vi "Access Any.vi"(8 "error in (no error)":errorcluster, 10 "Key":string, 11 "FlexWorktable in":refnum<class "FlexWorktable.lvclass">) -> (0 "error out":errorcluster, 1 "Type":string, 2 "Items out":T1, 3 "FlexWorktable out":refnum<class "FlexWorktable.lvclass">)   [LabVIEW 2022 SP3, in "FlexWorktable.lvclass"]
uses:
  FlexWorktable.lvclass
  Orient3d Class/Orient3d.lvclass
  Vec3d Class/Vec3d.lvclass
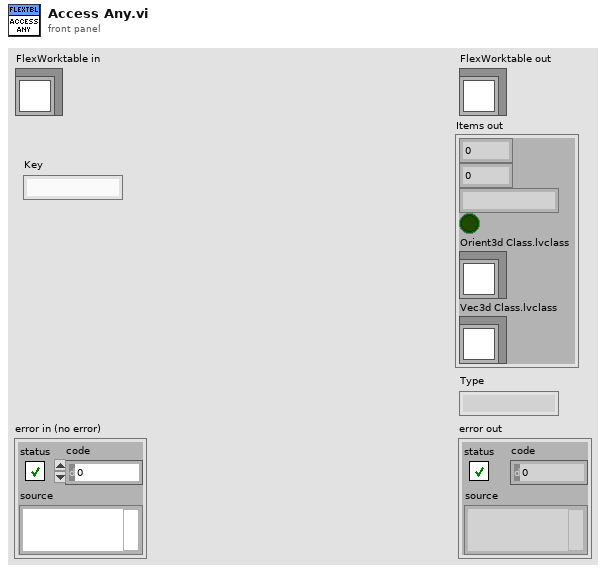
[diagram p1: front panel]
types:
  T1 = cluster{i32, dbl, string, bool, "Orient3d Class.lvclass":refnum<class "Orient3d.lvclass">, "Vec3d Class.lvclass":refnum<class "Vec3d.lvclass">}
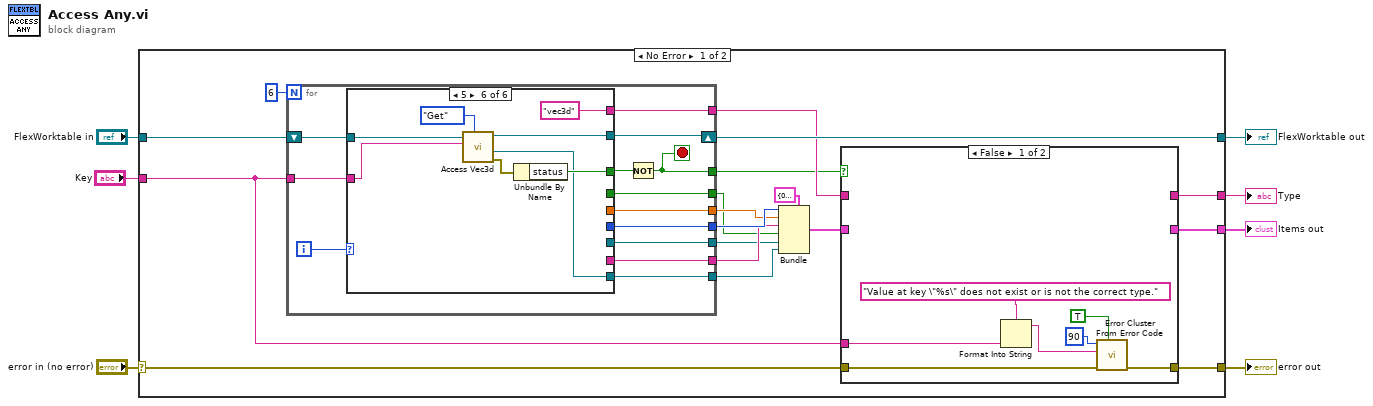
[diagram p0: block diagram]
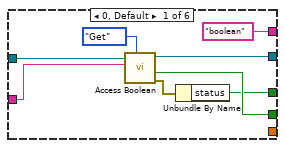
[diagram p3: hidden frame]
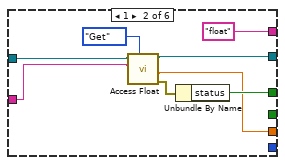
[diagram p4: hidden frame]
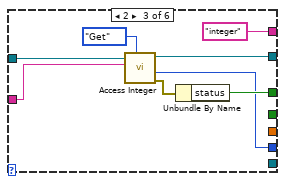
[diagram p5: hidden frame]
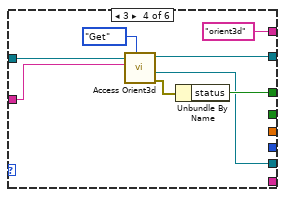
[diagram p6: hidden frame]
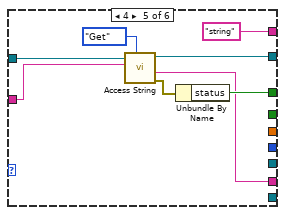
[diagram p7: hidden frame]
diagram:
  n1 = case shown="No Error" "error in (no error)" {
    selector: "error in (no error)" -> [w10 w98]
    tunnel: [w9 w98] -> w6
    tunnel: [w23 w97] -> w4
    tunnel: "FlexWorktable in" -> [w25 w97]
    tunnel: "Key" -> [w8 _]
    tunnel: [w11 _] -> w2
    tunnel: [w13 _] -> w1
    frame No Error {
      n2 = for {
        N: 6 -> [_]
        shift-right: [w45] -> w23
        shift-left: w25 -> [w47]
        tunnel: w8 -> [w46]
        tunnel: [w44] -> w18
        tunnel: [w42] -> w15
        tunnel: [w41] -> w14
        tunnel: [w40] -> w20
        tunnel: [w39] -> w21
        tunnel: [w38] -> w17
        tunnel: [w37] -> w19
        tunnel: [w36] -> w16
        i -> [w48]
        stop <- w41 stop-if-true
        n3 = case shown="5" w48 {
          tunnel: w47 -> [w56 w62 w72 w80 w88 w96]
          tunnel: w46 -> [w55 w58 w71 w79 w87 w95]
          tunnel: [w53 w61 w69 w77 w85 w93] -> w45
          tunnel: [w52 _ _ _ _ _] -> w44
          tunnel: [w50 w64 w67 w75 w83 w91] -> w43
          tunnel: ["boolean" "float" "integer" "orient3d" "string" "vec3d"] -> w42
          tunnel: [_ w60 _ _ _ _] -> w40
          tunnel: [_ _ w65 _ _ _] -> w39
          tunnel: [_ _ _ w73 _ _] -> w38
          tunnel: [_ _ _ _ w81 _] -> w37
          tunnel: [_ _ _ _ _ w89] -> w36
          frame 0, Default {
            n4 = call-dynamic "Access Boolean.vi"("Get/Set"=enum16{"Get", "Set"}."Get", "Key"=w55, "FlexWorktable in"=w56) -> ("error out"=w51:errorcluster, "Value out"=w52:bool, "FlexWorktable out"=w53:refnum<class "FlexWorktable.lvclass">)  [unwired: 6 in]
            n5 = Unbundle By Name(w51) -> ("status"=w50:bool)
          }
          frame 1 {
            n6 = call-dynamic "Access Float.vi"("Get/Set"=enum16{"Get", "Set"}."Get", "Key"=w58, "FlexWorktable in"=w62) -> ("error out"=w59:errorcluster, "Value out"=w60:dbl, "FlexWorktable out"=w61:refnum<class "FlexWorktable.lvclass">)  [unwired: 6 in]
            n7 = Unbundle By Name(w59) -> ("status"=w64:bool)
          }
          frame 2 {
            n8 = call-dynamic "Access Integer.vi"("Get/Set"=enum16{"Get", "Set"}."Get", "Key"=w71, "FlexWorktable in"=w72) -> ("error out"=w68:errorcluster, "Value out"=w65:i32, "FlexWorktable out"=w69:refnum<class "FlexWorktable.lvclass">)  [unwired: 6 in]
            n9 = Unbundle By Name(w68) -> ("status"=w67:bool)
          }
          frame 3 {
            n10 = call-dynamic "Access Orient3d.vi"("Get/Set"=enum16{"Get", "Set"}."Get", "Key"=w79, "FlexWorktable in"=w80) -> ("error out"=w76:errorcluster, "Value out"=w73:refnum<class "Orient3d.lvclass">, "FlexWorktable out"=w77:refnum<class "FlexWorktable.lvclass">)  [unwired: 6 in]
            n11 = Unbundle By Name(w76) -> ("status"=w75:bool)
          }
          frame 4 {
            n12 = call-dynamic "Access String.vi"("Get/Set"=enum16{"Get", "Set"}."Get", "Key"=w87, "FlexWorktable in"=w88) -> ("error out"=w84:errorcluster, "Value out"=w81:string, "FlexWorktable out"=w85:refnum<class "FlexWorktable.lvclass">)  [unwired: 6 in]
            n13 = Unbundle By Name(w84) -> ("status"=w83:bool)
          }
          frame 5 {
            n14 = call-dynamic "Access Vec3d.vi"("Get/Set"=enum16{"Get", "Set"}."Get", "Key"=w95, "FlexWorktable in"=w96) -> ("error out"=w92:errorcluster, "Value out"=w89:refnum<class "Vec3d.lvclass">, "FlexWorktable out"=w93:refnum<class "FlexWorktable.lvclass">)  [unwired: 6 in]
            n15 = Unbundle By Name(w92) -> ("status"=w91:bool)
          }
        }
        n16 = Not(x=w43) -> (.not. x?=w41:bool)
      }
      n17 = Bundle(cluster=T1 {0, 0.0, "", FALSE, "Orient3d Class.lvclass"=refnum, "Vec3d Class.lvclass"=refnum}, w21, w20, w19, w18, "Orient3d Class.lvclass"=w17, "Vec3d Class.lvclass"=w16) -> (w12:T1)
      n18 = case shown="False" w14 {
        tunnel: w15 -> [_ w35]
        tunnel: [_ w35] -> w13
        tunnel: w12 -> [_ w34]
        tunnel: [_ w34] -> w11
        tunnel: w10 -> [w28 w33]
        tunnel: [w27 w33] -> w9
        tunnel: w8 -> [w31 _]
        frame False {
          n19 = Format Into String(format string="Value at key \"%s\" does not exist or is not the correct type.", w31) -> (resulting string=w29:string)  [unwired: 2 in, 1 out]
          n20 = call <vilib>:"Error Cluster From Error Code.vi"("show call chain? (False)"=TRUE, "error in (no error)"=w28, "error message (\"\")"=w29, "error code (0)"=90) -> ("error out"=w27:errorcluster)  [unwired: 5 in]
        }
        frame True {
        }
      }
    }
    frame Error {
    }
  }
  "error out" <- w6
  "FlexWorktable out" <- w4
  "Type" <- w1
  "Items out" <- w2
